vi "PostBuildAction.vi"(5 "Files Generated by Build":path[](array[path]) caption="Vom Build erzeugte Dateien", 6 "Top Level/Always Included VIs":path[](array[path]) caption="Haupt-VIs/Immer enthaltene VIs", 7 "Destination Path":path caption="Zielpfad", 8 "error in (no error)":errorcluster caption="Fehler (Eingang, kein Fehler)", 9 "Target Name":string caption="Zielname", 10 "Build Specification Name":string caption="Name der Build-Spezifikation", 11 "Project Path":path caption="Projektpfad") -> (0 "error out":errorcluster caption="Fehler (Ausgang)")   [LabVIEW 2024]
uses:
  Typdefinitionen & Beschreibung/Post Build Action Zustand.ctl
  Typdefinitionen & Beschreibung/PostBuildActionCluster.ctl
  <vilib>/AppBuilder/AB_API_Simple/Get Build Specification Version (path).vi
  <vilib>/AppBuilder/AB_API_Simple/Set Build Specification Version (path).vi
  kernel32.dll
  <vilib>/AppBuilder/AB_API_Simple/NI_App_Builder_API.lvlib
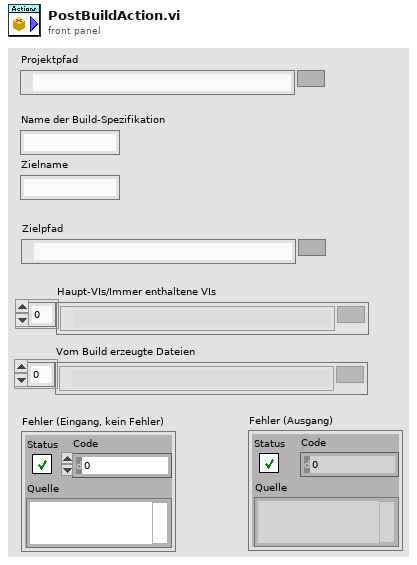
[diagram p1: front panel]
types:
  T1 = typedef "PostBuildActionCluster.ctl" = cluster{"Major":string, "Minor":string, "Fix":string, "Build":string, "USB-Stick vorhanden?":bool, "USB-Stick Name":string}
  T2 = typedef "Post Build Action Zustand.ctl" = enum16{"Version auslesen und USB-Stick suchen", "Archiv erstellen", "Auf USB-Stick kopieren"}
  T3 = typedef "NI_App_Builder_API.lvlib/Build Specification Version.ctl" = cluster{"Major":u16, "Minor":u16, "Fix":u16, "Build":u16}
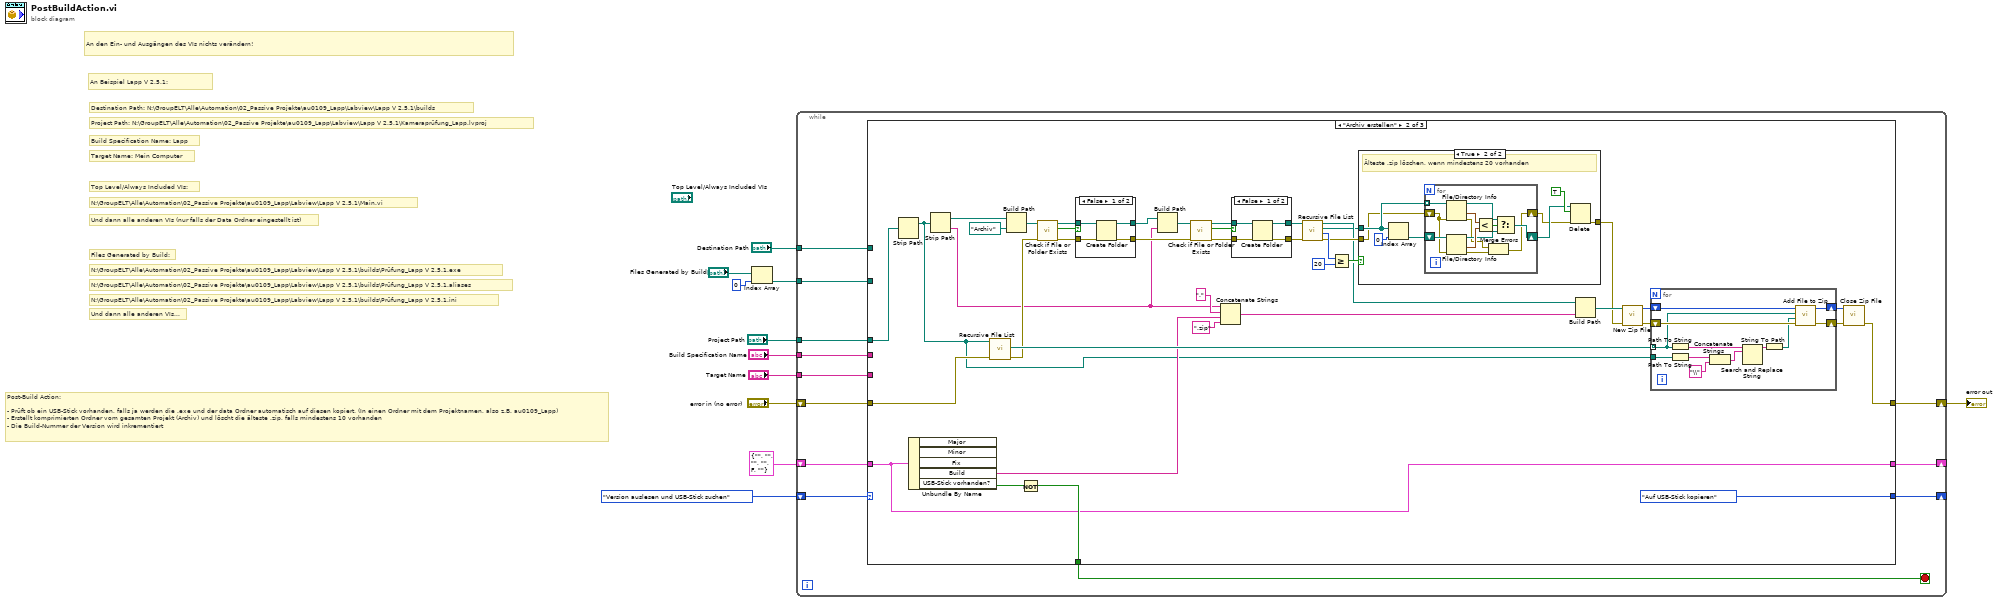
[diagram p0: block diagram]
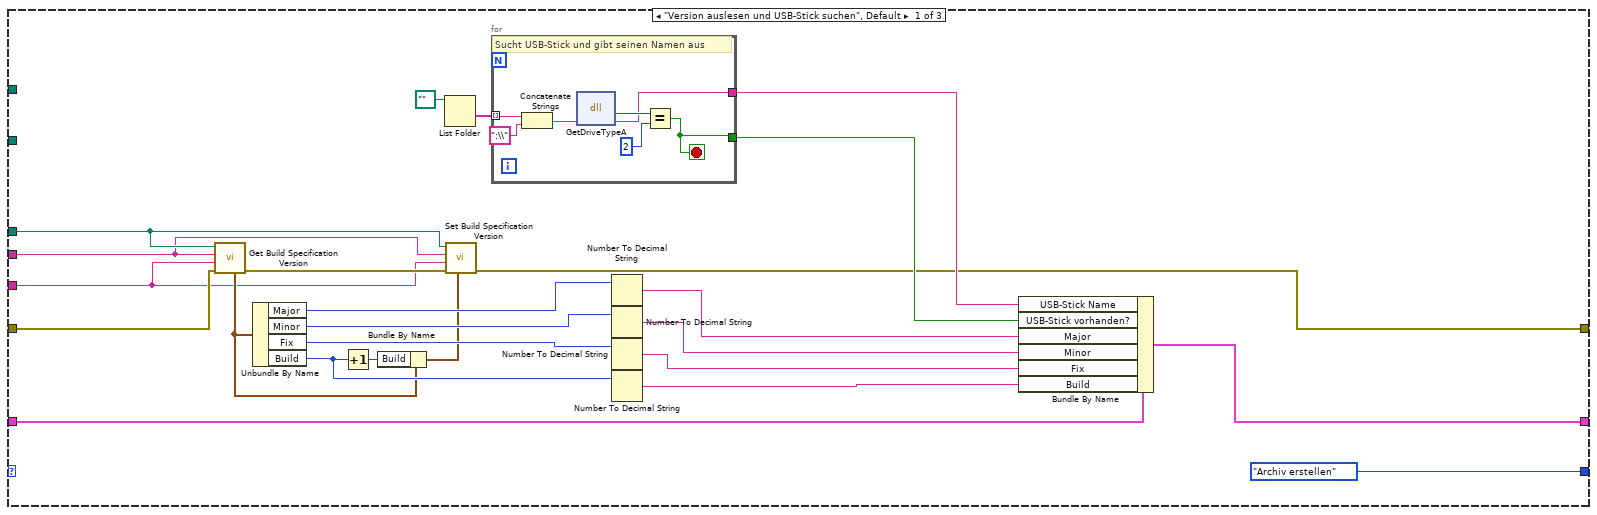
[diagram p2: hidden frame]
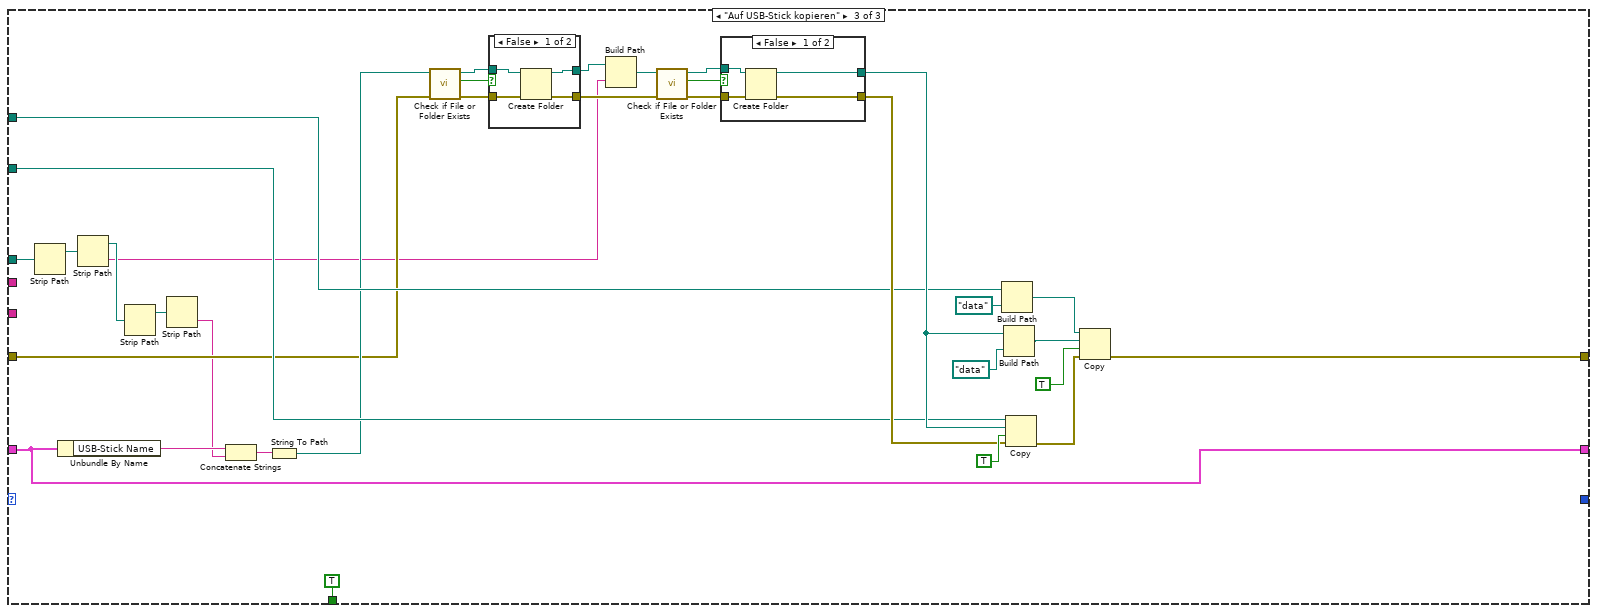
[diagram p6: hidden frame]
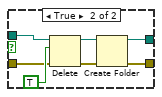
[diagram p7: hidden frame]
diagram:
  # "Post-Build Action:\n\n- Prüft ob ein USB-Stick vorhanden, falls ja werden die .exe und der data Ordner automatisch auf diesen kopiert. (In einen Ordner mit dem Projektnamen, also z.B. au0109_Lapp)\n- Erstellt komprimierten Ordner vom gesamten Projekt (Archiv) und löscht die älteste .zip, falls mindestens 10 vorhanden\n- Die Build-Nummer der Version wird inkrementiert"
  # "An den Ein- und Ausgängen des VIs nichts verändern!"
  # "Files Generated by Build:"
  # "N:\\GroupELT\\Alle\\Automation\\02_Passive Projekte\\au0109_Lapp\\Labview\\Lapp V 2.5.1\\Main.vi"
  # "Top Level/Always Included VIs:"
  # "Target Name: Mein Computer"
  # "Build Specification Name: Lapp"
  # "Project Path: N:\\GroupELT\\Alle\\Automation\\02_Passive Projekte\\au0109_Lapp\\Labview\\Lapp V 2.5.1\\Kameraprüfung_Lapp.lvproj"
  # "Destination Path: N:\\GroupELT\\Alle\\Automation\\02_Passive Projekte\\au0109_Lapp\\Labview\\Lapp V 2.5.1\\builds"
  # "An Beispiel Lapp V 2.5.1:"
  # "Und dann alle anderen VIs (nur falls der Data Ordner eingestellt ist)"
  # "Und dann alle anderen VIs..."
  # "N:\\GroupELT\\Alle\\Automation\\02_Passive Projekte\\au0109_Lapp\\Labview\\Lapp V 2.5.1\\builds\\Prüfung_Lapp V 2.5.1.ini"
  # "N:\\GroupELT\\Alle\\Automation\\02_Passive Projekte\\au0109_Lapp\\Labview\\Lapp V 2.5.1\\builds\\Prüfung_Lapp V 2.5.1.aliases"
  # "N:\\GroupELT\\Alle\\Automation\\02_Passive Projekte\\au0109_Lapp\\Labview\\Lapp V 2.5.1\\builds\\Prüfung_Lapp V 2.5.1.exe"
  n1 = Index Array(array="Files Generated by Build", index=0) -> (element=w3:path)
  n2 = while {
    shift-right: [w22] -> _
    shift-left: Post_Build_Action_Zustand."Version auslesen und USB-Stick suchen" -> [w23]
    tunnel: "Build Specification Name" -> [w19]
    tunnel: "Target Name" -> [w18]
    shift-right: [w14] -> w2
    shift-left: "error in (no error)" -> [w17]
    tunnel: "Project Path" -> [w16]
    shift-right: [w15] -> _
    shift-left: T1 {"Major"="", "Minor"="", "Fix"="", "Build"="", "USB-Stick vorhanden?"=FALSE, "USB-Stick Name"=""} -> [w21]
    tunnel: "Destination Path" -> [w12]
    tunnel: w3 -> [w13]
    stop <- w20 stop-if-true
    n3 = case shown="\"Archiv erstellen\"" w23 {
      tunnel: [Post_Build_Action_Zustand."Archiv erstellen" Post_Build_Action_Zustand."Auf USB-Stick kopieren" _] -> w22
      tunnel: w21 -> [w43 w69 w145]
      tunnel: [_ w93 TRUE ("USB-Stick vorhanden?")] -> w20
      tunnel: w19 -> [w25 _ _]
      tunnel: w18 -> [w26 _ _]
      tunnel: w17 -> [w46 w79 w146]
      tunnel: w16 -> [w27 w86 w152]
      tunnel: [w40 w69 w145] -> w15
      tunnel: [w24 w87 w158] -> w14
      tunnel: w13 -> [_ _ w151]
      tunnel: w12 -> [_ _ w150]
      frame "Version auslesen und USB-Stick suchen", Default {
        n4 = call-poly <vilib>:"Get Build Specification Version.vi"("error in (no error)"=w46, "Name of target (My Computer)"=w26, "Name of build specification"=w25, "Path to project"=w27) -> ("error out"=w29:errorcluster, "Build Specification Version"=w28:T3)  [unwired: 6 in]
        n5 = Unbundle By Name(w28) -> ("Major"=w39:u16, "Minor"=w38:u16, "Fix"=w37:u16, "Build"=w30:u16)
        n6 = Increment(x=w30) -> (x+1=w32:u16)
        n7 = Bundle By Name(cluster=w28, "Build"=w32) -> (w31:T3)
        n8 = List Folder(path=path "" ("Pfad")) -> (folder names=w45:string[])  [unwired: 3 in, 3 out]
        n9 = call-poly <vilib>:"Set Build Specification Version.vi"("Build Specification Version"=w31, "error in (no error)"=w29, "Name of target (My Computer)"=w26, "Name of build specification"=w25, "Path to project"=w27) -> ("error out"=w24:errorcluster)  [unwired: 6 in]
        n10 = for {
          tunnel: w45 -> [w54] mode=indexing
          tunnel: [w49] -> w42
          tunnel: [w48] -> w41
          stop <- w48 stop-if-true
          # "Sucht USB-Stick und gibt seinen Namen aus"
          n11 = Concatenate Strings(w54, ":\\" ("String")) -> (w52:string)
          n12 = dll-call lib="kernel32.dll" fn="GetDriveTypeA"("arg1"=w52) -> ("Ausgabetyp"=w51:u32, "arg1"=w49:string)  [unwired: 3 in, 2 out]
          n13 = Equal?(x=w51, y=u32 2) -> (x = y?=w48:bool)
        }
        n14 = Number To Decimal String(number=w39) -> (decimal integer string=w36:string)  [unwired: 1 in]
        n15 = Number To Decimal String(number=w38) -> (decimal integer string=w35:string)  [unwired: 1 in]
        n16 = Number To Decimal String(number=w37) -> (decimal integer string=w34:string)  [unwired: 1 in]
        n17 = Number To Decimal String(number=w30) -> (decimal integer string=w33:string)  [unwired: 1 in]
        n18 = Bundle By Name(cluster=w43, "USB-Stick Name"=w42, "USB-Stick vorhanden?"=w41, "Major"=w36, "Minor"=w35, "Fix"=w34, "Build"=w33) -> (w40:T1)
      }
      frame "Archiv erstellen" {
        n19 = Strip Path(path=w86) -> (stripped path=w68:path)  [unwired: 1 out]
        n20 = Unbundle By Name(w69) -> ("Build"=w70:string, "USB-Stick vorhanden?"=w94:bool)  [unwired: 3 out]
        n21 = Strip Path(path=w68) -> (stripped path=w77:path, name=w55:string)
        n22 = call <vilib>:"Recursive File List.vi"("error in (no error)"=w79, "Folder Path"=w68) -> ("error out"=w78:errorcluster, "All Files in Dir"=w80:path[])  [unwired: 5 in, 3 out]
        n23 = Build Path(base path=w77, name or relative path=path "Archiv" ("Name oder relativer Pfad")) -> (appended path=w84:path)
        n24 = Not(x=w94) -> (.not. x?=w93:bool)
        n25 = call <vilib>:"Check if File or Folder Exists.vi"("error in (no error)"=w78, "path"=w84) -> ("error out"=w85:errorcluster, "file or folder exists?"=w82:bool, "dup path"=w81:path)  [unwired: 7 in]
        n26 = case shown="False" w82 {
          tunnel: w81 -> [w126 w128]
          tunnel: [w125 w128] -> w76
          tunnel: w85 -> [w124 w127]
          tunnel: [w123 w127] -> w74
          frame False {
            n27 = Create Folder(path (use dialog)=w126, error in=w124) -> (created path=w125:path, error out=w123:errorcluster)  [unwired: 1 in, 1 out]
          }
          frame True {
          }
        }
        n28 = Build Path(base path=w76, name or relative path=w55) -> (appended path=w75:path)
        n29 = call <vilib>:"Check if File or Folder Exists.vi"("error in (no error)"=w74, "path"=w75) -> ("error out"=w65:errorcluster, "file or folder exists?"=w66:bool, "dup path"=w67:path)  [unwired: 7 in]
        n30 = Concatenate Strings(w55, "." ("String"), w70, ".zip" ("String")) -> (w71:string)
        n31 = case shown="False" w66 {
          tunnel: w67 -> [w120 w122]
          tunnel: [w119 w122] -> w63
          tunnel: w65 -> [w118 w121]
          tunnel: [w117 w121] -> w64
          frame False {
            n32 = Create Folder(path (use dialog)=w120, error in=w118) -> (created path=w119:path, error out=w117:errorcluster)  [unwired: 1 in, 1 out]
          }
          frame True {
          }
        }
        n33 = call <vilib>:"Recursive File List.vi"("error in (no error)"=w64, "Folder Path"=w63) -> ("error out"=w59:errorcluster, "Number of Files"=w62:i32, "All Files in Dir"=w57:path[], "dup Folder Path"=w58:path)  [unwired: 5 in, 1 out]
        n34 = Greater Or Equal?(x=w62, y=20) -> (x >= y?=w60:bool)
        n35 = case shown="True" w60 {
          tunnel: w59 -> [w96 w98]
          tunnel: w57 -> [_ w99]
          tunnel: [w96 w102] -> w56
          frame False {
          }
          frame True {
            # "Älteste .zip löschen, wenn mindestens 20 vorhanden"
            n36 = Index Array(array=w99, index=0) -> (element=w101:path)
            n37 = for {
              tunnel: w99 -> [w112] mode=indexing
              shift-right: [w116] -> w100
              shift-left: w101 -> [w111]
              shift-right: [w105] -> w97
              shift-left: w98 -> [w108]
              n38 = File/Directory Info(path=w112, error in=w108) -> (path out=w113:path, last mod=w114:timestamp, error out=w106:errorcluster)  [unwired: 4 out]
              n39 = File/Directory Info(path=w111, error in=w108) -> (path out=w109:path, last mod=w110:timestamp, error out=w107:errorcluster)  [unwired: 4 out]
              n40 = Less?(x=w114, y=w110) -> (x < y?=w115:bool)
              n41 = Merge Errors(w106, w107) -> (w105:errorcluster)
              n42 = Select(t=w113, s=w115, f=w109) -> (s? t:f=w116:path)
            }
            n43 = Delete(path (use dialog)=w100, entire hierarchy (F)=TRUE, error in=w97) -> (error out=w102:errorcluster)  [unwired: 2 in, 2 out]
          }
        }
        n44 = Build Path(base path=w58, name or relative path=w71) -> (appended path=w88:path)
        n45 = call <vilib>:"New Zip File.vi"("error in (no error)"=w56, "target"=w88) -> ("error out"=w92:errorcluster, "zip file out"=w91:i64)  [unwired: 3 in, 1 out]
        n46 = for {
          shift-right: [w139] -> w89
          shift-left: w92 -> [w138]
          shift-right: [w140] -> w90
          shift-left: w91 -> [w137]
          tunnel: w80 -> [w135] mode=indexing
          tunnel: w68 -> [w136]
          n47 = Path To String(path=w135) -> (string=w132:string)
          n48 = Path To String(path=w136) -> (string=w133:string)
          n49 = Concatenate Strings(w133, "\\" ("String")) -> (w131:string)
          n50 = Search and Replace String(input string=w132, search string=w131) -> (result string=w130:string)  [unwired: 6 in, 3 out]
          n51 = String To Path(string=w130) -> (path=w129:path)
          n52 = call <vilib>:"Add File to Zip.vi"("error in (no error)"=w138, "destination path in zip"=w129, "source file path"=w135, "zip file in"=w137) -> ("error out"=w139:errorcluster, "zip file out"=w140:i64)  [unwired: 6 in]
        }
        n53 = call <vilib>:"Close Zip File.vi"("error in (no error)"=w89, "zip file in"=w90) -> ("error out"=w87:errorcluster)  [unwired: 5 in]
      }
      frame "Auf USB-Stick kopieren" {
        n54 = Strip Path(path=w152) -> (stripped path=w153:path)  [unwired: 1 out]
        n55 = Unbundle By Name(w145) -> ("USB-Stick Name"=w148:string)
        n56 = Strip Path(path=w153) -> (stripped path=w144:path, name=w141:string)
        n57 = Strip Path(path=w144) -> (stripped path=w143:path)  [unwired: 1 out]
        n58 = Strip Path(path=w143) -> (name=w142:string)  [unwired: 1 out]
        n59 = Concatenate Strings(w148, w142) -> (w149:string)
        n60 = String To Path(string=w149) -> (path=w147:path)
        n61 = call <vilib>:"Check if File or Folder Exists.vi"("error in (no error)"=w146, "path"=w147) -> ("error out"=w157:errorcluster, "file or folder exists?"=w160:bool, "dup path"=w161:path)  [unwired: 7 in]
        n62 = case shown="False" w160 {
          tunnel: w161 -> [w188 w190]
          tunnel: [w187 w190] -> w163
          tunnel: w157 -> [w186 w189]
          tunnel: [w185 w189] -> w156
          frame False {
            n63 = Create Folder(path (use dialog)=w188, error in=w186) -> (created path=w187:path, error out=w185:errorcluster)  [unwired: 1 in, 1 out]
          }
          frame True {
          }
        }
        n64 = Build Path(base path=w163, name or relative path=w141) -> (appended path=w162:path)
        n65 = call <vilib>:"Check if File or Folder Exists.vi"("error in (no error)"=w156, "path"=w162) -> ("error out"=w155:errorcluster, "file or folder exists?"=w164:bool, "dup path"=w165:path)  [unwired: 7 in]
        n66 = case shown="False" w164 {
          tunnel: w165 -> [w177 w183]
          tunnel: [w176 w181] -> w159
          tunnel: w155 -> [w175 w180]
          tunnel: [w174 w178] -> w154
          frame False {
            n67 = Create Folder(path (use dialog)=w177, error in=w175) -> (created path=w176:path, error out=w174:errorcluster)  [unwired: 1 in, 1 out]
          }
          frame True {
            n68 = Delete(path (use dialog)=w183, entire hierarchy (F)=TRUE ("Gesamte Hierarchie (F)"), error in=w180) -> (deleted path=w182:path, error out=w179:errorcluster)  [unwired: 2 in, 1 out]
            n69 = Create Folder(path (use dialog)=w182, error in=w179) -> (created path=w181:path, error out=w178:errorcluster)  [unwired: 1 in, 1 out]
          }
        }
        n70 = Build Path(base path=w150, name or relative path=path "data" ("Name oder relativer Pfad")) -> (appended path=w170:path)
        n71 = Build Path(base path=w159, name or relative path=path "data" ("Zielpfad (Dialog verwenden)")) -> (appended path=w166:path)
        n72 = Copy(8:w154, 9:TRUE ("Überschreiben (F)"), 10:w159, 11:w151) -> (0:w168:errorcluster)  [unwired: 1 in, 2 out]
        n73 = Copy(8:w168, 9:TRUE ("Überschreiben (F)"), 10:w166, 11:w170) -> (0:w158:errorcluster)  [unwired: 1 in, 2 out]
      }
    }
  }
  "error out" <- w2
